vi "Register as Listener.vi"(8 "error in (no error)":errorcluster, 11 "Example Actor in":refnum<class "Example Actor.lvclass">) -> (0 "error out":errorcluster, 3 "Example Actor out":refnum<class "Example Actor.lvclass">)   [LabVIEW 2016, in "Example Actor.lvclass"]
doc: "--\nCopyright © 2017 Composed SystemsI All rights reserved.\n\nAuthor: Jon McBee <jon.mcbee@composed.io>\n\nThis library is provided \"AS IS\" ,WITHOUT WARRANTIES OR\nCONDITIONS OF ANY KIND, either express or implied.\n\nComposed Systems -- composed.io\n\nStream 0.0.1.1\nJon McBee - Composed Systems\nCopyright (c) 2017, Composed Systems"
uses:
  <userlib>/Composed Systems/Stream/Mediator/Example/Example Actor/Example Actor.lvclass
  C:/Program Files (x86)/National Instruments/LabVIEW 2016/vi.lib/ActorFramework/Actor/Actor.lvclass
  <userlib>/Composed Systems/Stream/Mediator/Example/Example Actor Messages/Sample Actor Data Msg/Sample Actor Data Msg.lvclass
  C:/Program Files (x86)/National Instruments/LabVIEW 2016/user.lib/Composed Systems/Stream/Mediator/Classes/Message AF Mediator/Message AF Mediator.lvclass
  <vilib>/ActorFramework/Actor/Actor.lvclass/Actor.ctl
  <vilib>/ActorFramework/Message Enqueuer/Message Enqueuer.lvclass/Message Enqueuer.ctl
  <userlib>/Composed Systems/Stream/Mediator/Example/Example Actor/Example Actor.lvclass/Example Actor.ctl
  <vilib>/ActorFramework/Message Enqueuer/Init from Existing Queue.vi
  <userlib>/Composed Systems/Stream/Mediator/Classes/Message Transport Actor Framework/Message Transport Actor Framework.lvclass
  C:/Program Files (x86)/National Instruments/LabVIEW 2016/user.lib/Composed Systems/Stream/Mediator/Classes/Message Transport Interface/Message Transport Interface.lvclass
  <vilib>/ActorFramework/Message Enqueuer/Message Enqueuer.lvclass
  <userlib>/Composed Systems/Stream/Mediator/Classes/Message Broker Interface Ref/Message Broker Interface Ref.lvclass
  <vilib>/ActorFramework/Actor/Actor.lvclass
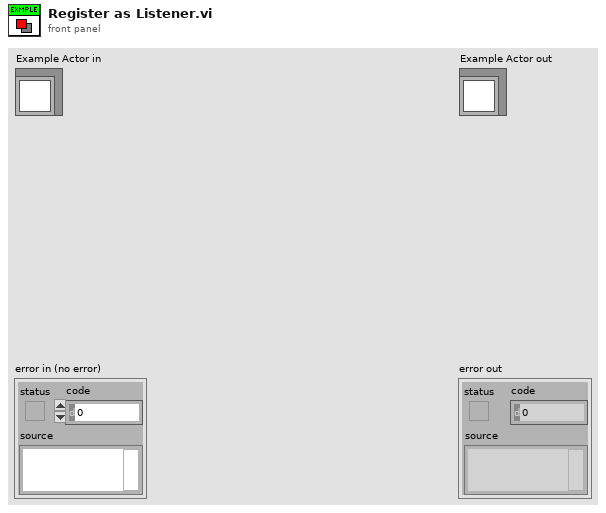
[diagram p1: front panel]
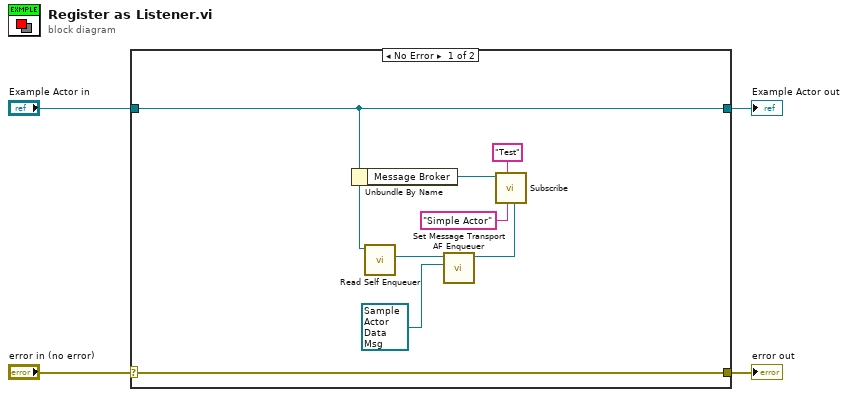
[diagram p0: block diagram]
diagram:
  n1 = case shown="No Error" "error in (no error)" {
    selector: "error in (no error)" -> [w12 w14]
    tunnel: [w12 w14] -> w3
    tunnel: [w6 w13] -> w1
    tunnel: "Example Actor in" -> [w6 w13]
    frame No Error {
      n2 = Unbundle By Name(w6) -> ("Message Broker"=w10:refnum<class "Message Broker Interface Ref.lvclass">)
      n3 = call <vilib>:"Read Self Enqueuer.vi"("Actor"=w6) -> ("Self Enqueuer"=w8:refnum<class "Message Enqueuer.lvclass">)  [unwired: 10 in]
      n4 = call <userlib>:"Set Message Transport AF Enqueuer.vi"("Message AF Mediator"=refnum<class "Sample Actor Data Msg.lvclass"> refnum ("Sample Actor Data Msg.lvclass"), "Actor's Enqueuer"=w8) -> ("Message Transport Actor Framework out"=w7:refnum<class "Message Transport Actor Framework.lvclass">)  [unwired: 8 in, 1 out]
      n5 = call-dynamic "Subscribe.vi"("Message Transport Interface"=w7, "Subscriber Name"="Simple Actor", "Topic Name"="Test", "Message Broker Interface TAP in"=w10) -> ()  [unwired: 5 in, 3 out]
    }
    frame Error {
    }
  }
  "error out" <- w3
  "Example Actor out" <- w1
